vi "Data_Write_Single.vi"(7 "wfm info":T2, 8 "error in (no error)":errorcluster, 10 "QMH ICR Cluster":T1, 11 "data":i16[](array[numeric])) -> (0 "error out":errorcluster, 3 "data":i16[](array[numeric]))   [LabVIEW 2024]
doc: "This VI writes a raw dataset to a disk file with the following format :\n- number of points = one value (I16)\n- data = number of points values (I16)\n- 1/sample rate, i.e. time step = one value (DBL)\n- vertical range = one value (DBL)\n- offset = one value (DBL)\nCalibrated data are obtained with : data * vertical range + offset\n\nThe file naming convention is :\nyyyy_mm_dd_xxx.A00 for the first acqusisition,\nyyyy_mm_dd_xxx.B00 for the second, etc."
uses:
  controls/QMH_ICR_Cluster.ctl
  controls/HARDWARE_Resources.ctl
  controls/PROCESSING_Inputs.ctl
  controls/LOOPS_Inputs.ctl
  controls/OPO_Inputs.ctl
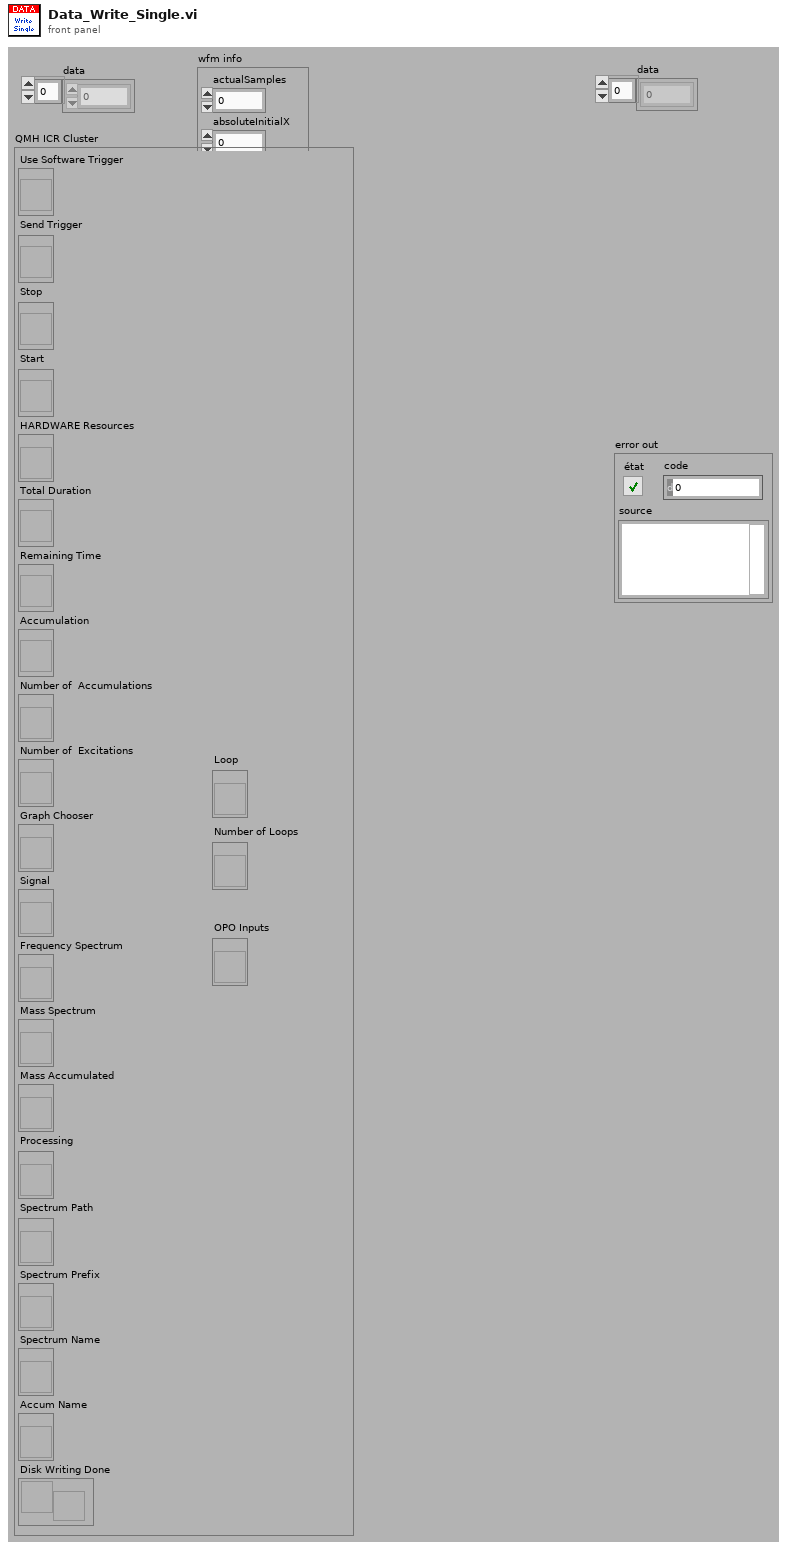
[diagram p1: front panel]
types:
  T1 = typedef "QMH_ICR_Cluster.ctl" = cluster{"Use Software Trigger":refnum<vi>, "Send Trigger":refnum<vi>, "Stop":refnum<vi>, "Start":refnum<vi>, "HARDWARE Resources":refnum<vi>, "Total Duration":refnum<vi>, "Remaining Time":refnum<vi>, "Accumulation":refnum<vi>, "Number of  Accumulations":refnum<vi>, "Number of  Excitations":refnum<vi>, "Graph Chooser":refnum<vi>, "Signal":refnum<vi>, "Frequency Spectrum":refnum<vi>, "Mass Spectrum":refnum<vi>, "Mass Accumulated":refnum<vi>, "Processing":refnum<vi>, "Spectrum Path":refnum<vi>, "Spectrum Prefix":refnum<vi>, "Spectrum Name":refnum<vi>, "Accum Name":refnum<vi>, "Disk Writing Done":refnum<notifier>, "Loop":refnum<vi>, "Number of Loops":refnum<vi>, "OPO Inputs":refnum<vi>}
  T2 = cluster{"actualSamples":i32, "absoluteInitialX":dbl, "relativeInitialX":dbl, "xIncrement":dbl, "offset":dbl, "gain":dbl, "reserved1":dbl, "reserved2":dbl}
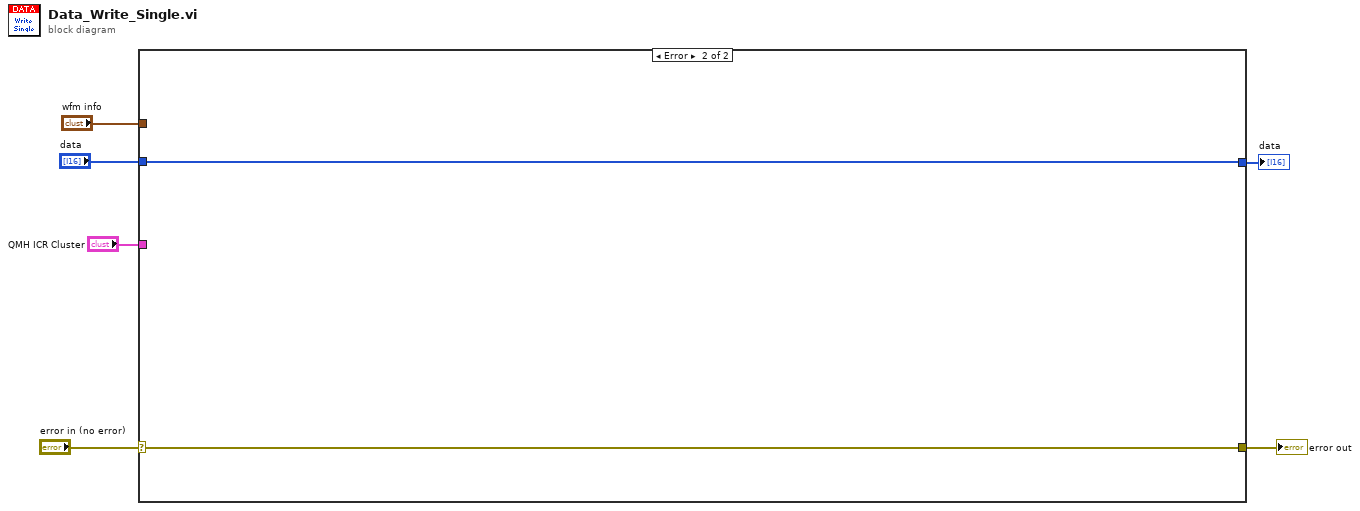
[diagram p0: block diagram]
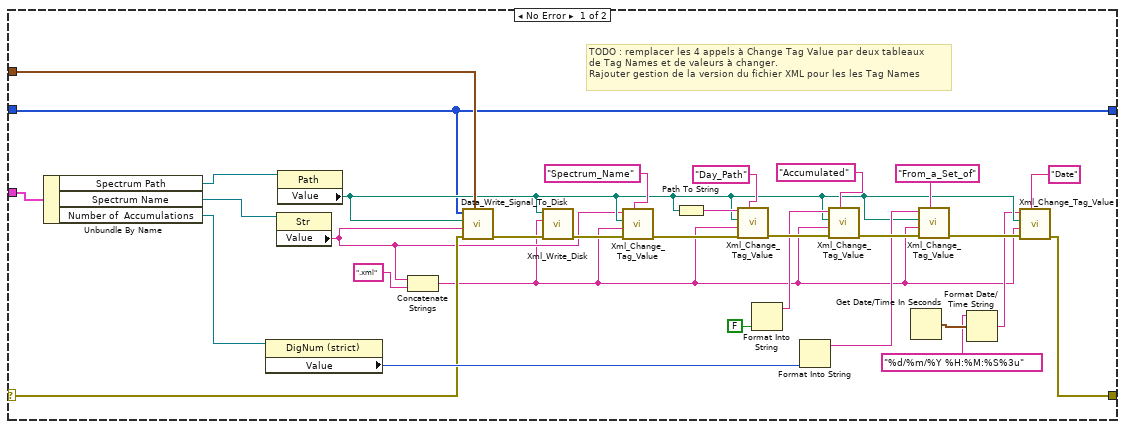
[diagram p2: hidden frame]
diagram:
  n1 = case shown="Error" "error in (no error)" {
    selector: "error in (no error)" -> [w19 w39]
    tunnel: [w16 w39] -> w5
    tunnel: "QMH ICR Cluster" -> [w21 _]
    tunnel: "wfm info" -> [w35 _]
    tunnel: "data" -> [w7 w38]
    tunnel: [w7 w38] -> w1
    frame No Error {
      # "TODO : remplacer les 4 appels à Change Tag Value par deux tableaux\nde Tag Names et de valeurs à changer.\nRajouter gestion de la version du fichier XML pour les les Tag Names"
      n2 = Unbundle By Name(w21) -> ("Spectrum Path"=w37:refnum<vi>, "Spectrum Name"=w36:refnum<vi>, "Number of  Accumulations"=w29:refnum<vi>)
      n3 = property class="DigNum (strict)"(reference=w29) -> ("Value"=w20:i16)  [unwired: 1 in, 2 out]
      n4 = property class="Str"(reference=w36) -> ("Value"=w11:string)  [unwired: 1 in, 2 out]
      n5 = property class="Path"(reference=w37) -> ("Value"=w15:path)  [unwired: 1 in, 2 out]
      n6 = Concatenate Strings(w11, ".xml" ("chaîne")) -> (w9:string)
      n7 = call "Data_Write_Signal_To_Disk.vi"("wfm info"=w35, "error in (no error)"=w19, "filename"=w11, "path"=w15, "data"=w7) -> ("error out"=w34:errorcluster)  [unwired: 6 in]
      n8 = call "Xml_Write_Disk.vi"("error in (no error)"=w34, "XML Name"=w9, "Spectrum Path"=w15) -> ("error out"=w33:errorcluster)  [unwired: 7 in, 1 out]
      n9 = call "Xml_Change_Tag_Value.vi"("Tag Name"="Spectrum_Name" ("New Value"), "error in (no error)"=w33, "XML Filename"=w9, "XML Path"=w15, "New Value"=w11) -> ("error out"=w32:errorcluster)  [unwired: 4 in, 2 out]
      n10 = Path To String(path=w15) -> (string=w25:string)
      n11 = call "Xml_Change_Tag_Value.vi"("Tag Name"="Day_Path", "error in (no error)"=w32, "XML Filename"=w9, "XML Path"=w15, "New Value"=w25) -> ("error out"=w31:errorcluster)  [unwired: 4 in, 2 out]
      n12 = Format Into String(FALSE ("entrée 1")) -> (resulting string=w24:string)  [unwired: 3 in, 1 out]
      n13 = Format Into String(w20) -> (resulting string=w23:string)  [unwired: 3 in, 1 out]
      n14 = call "Xml_Change_Tag_Value.vi"("Tag Name"="Accumulated" ("New Value"), "error in (no error)"=w31, "XML Filename"=w9, "XML Path"=w15, "New Value"=w24) -> ("error out"=w30:errorcluster)  [unwired: 4 in, 2 out]
      n15 = Get Date/Time In Seconds() -> (seconds since 1Jan1904=w14:timestamp)
      n16 = call "Xml_Change_Tag_Value.vi"("Tag Name"="From_a_Set_of", "error in (no error)"=w30, "XML Filename"=w9, "XML Path"=w15, "New Value"=w23) -> ("error out"=w17:errorcluster)  [unwired: 4 in, 2 out]
      n17 = Format Date/Time String(time format string (%c)="%d/%m/%Y %H:%M:%S%3u" ("chaîne de format de l'heure (%c)"), seconds (now)=w14) -> (date/time string=w12:string)  [unwired: 1 in]
      n18 = call "Xml_Change_Tag_Value.vi"("Tag Name"="Date", "error in (no error)"=w17, "XML Filename"=w9, "XML Path"=w15, "New Value"=w12) -> ("error out"=w16:errorcluster)  [unwired: 4 in, 2 out]
    }
    frame Error {
    }
  }
  "error out" <- w5
  "data" <- w1
